vi "温度计.vi"() -> ()   [LabVIEW 2020]
panel:
  in  "开关":bool
  out "报警":bool
  in  "数值":dbl
  out "电压(mV)":T1 scale=0.0..1000.0
  out "温度计":dbl(slide) scale=0.0..100.0
  # "虚拟温度计"
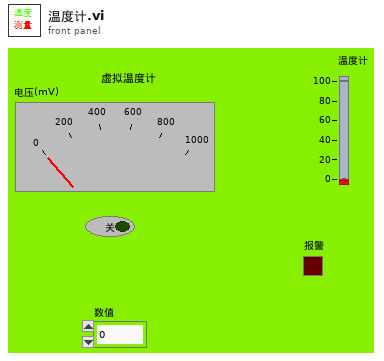
[diagram p1: front panel]
types:
  T1 = typedef "控件 1.ctl" = dbl
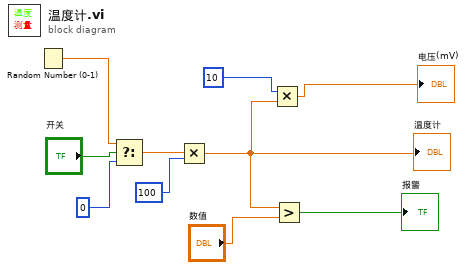
[diagram p0: block diagram]
diagram:
  n1 = Random Number (0-1)() -> (number: 0 to 1=w3:dbl)
  n2 = Select(t=w3, s="开关", f=0) -> (s? t:f=w8:dbl)
  n3 = Multiply(x=w8, y=100) -> (x*y=w4:dbl)
  "温度计" <- w4
  n4 = Multiply(x=10, y=w4) -> (x*y=→"电压(mV)":dbl)
  n5 = Greater?(x=w4, y="数值") -> (0:→"报警":bool)
